vi "BuildDefaultPlaylist.vi"() -> ()   [LabVIEW 2010]
panel:
  out "Table Control 2":string[][](table)
  out "Table Control":string[][](table)
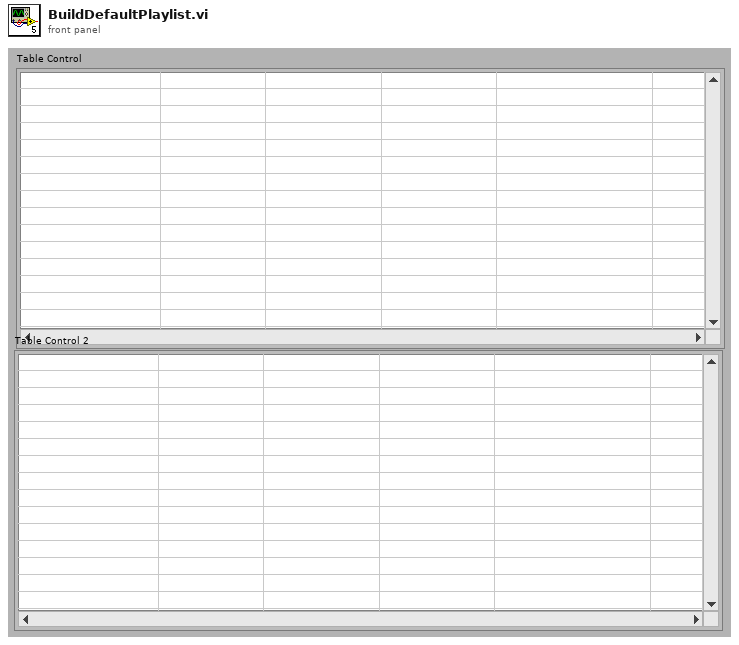
[diagram p1: front panel]
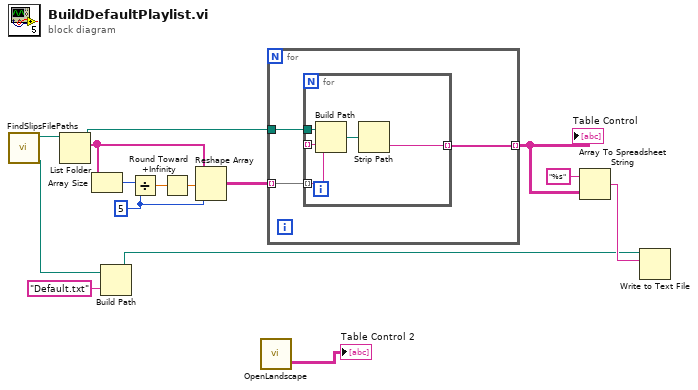
[diagram p0: block diagram]
diagram:
  w11 = 5 ("y")
  n1 = call "FindSlipsFilePaths.vi"() -> ("Playlists"=w2:path, "Slides"=w1:path)  [unwired: 2 in, 3 out]
  n2 = List Folder(path=w1) -> (path out=w15:path, filenames=w14:string[])  [unwired: 3 in, 2 out]
  n3 = Array Size(array=w14) -> (size(s)=w13:i32)
  n4 = Build Path(base path=w2, name or relative path="Default.txt") -> (appended path=w4:path)
  n5 = Divide(x=w13, y=w11) -> (x/y=w12:dbl)
  n6 = Round Toward +Infinity(x=w12) -> (ceil(x): smallest int >= x=w10:dbl)
  n7 = Reshape Array(w14, w10, w11) -> (w9:string[][])
  n8 = call "OpenLandscape.vi"() -> ("Landscape"=→"Table Control 2":string[][])  [unwired: 1 in, 1 out]
  n9 = for {
    tunnel: w15 -> [w18]
    tunnel: w9 -> [w17] mode=indexing
    tunnel: [w16] -> w8 mode=indexing
    n10 = for {
      tunnel: w18 -> [w22]
      tunnel: [w21] -> _ mode=indexing
      tunnel: w17 -> [w21] mode=indexing
      tunnel: [w19] -> w16 mode=indexing
      n11 = Build Path(base path=w22, name or relative path=w21) -> (appended path=w20:path)
      n12 = Strip Path(path=w20) -> (name=w19:string)  [unwired: 1 out]
    }
  }
  "Table Control" <- w8
  n13 = Array To Spreadsheet String(array=w8, 3:"%s" ("format string")) -> (spreadsheet string=w5:string)  [unwired: 1 in]
  n14 = Write to Text File(file (use dialog)=w4, text=w5) -> ()  [unwired: 2 in, 3 out]
